vi "CEF_error generator.vi"(4 "concatenate (F)":bool, 5 "error (T)":bool=TRUE, 6 "error in":errorcluster, 7 "source":string="error generator.vi", 8 "append error message":string, 9 "error code (0)":i32) -> (0 "error out":errorcluster)   [LabVIEW 2025, in "CEF.lvlib"]
doc: "Converts an error or warning code to an error cluster. This VI is useful when you receive a return value from a shared library call or when you return user-defined error codes.Copyright 2017 National Instruments Corporation\n\nLicensed under the Apache License, Version 2.0 (the \"License\"); you may not use this file except in compliance with the License. You may obtain a copy of the License at http://www.apache.org/licenses/LICENSE-2.0\nUnless required by applicable law or agreed to in writing, software distributed under the License is distributed on an \"AS IS\" BASIS, WITHOUT WARRANTIES OR CONDITIONS OF ANY KIND, either express or implied. See the License for the specific language governing permissions and limitations under the License."
uses:
  CEF.lvlib
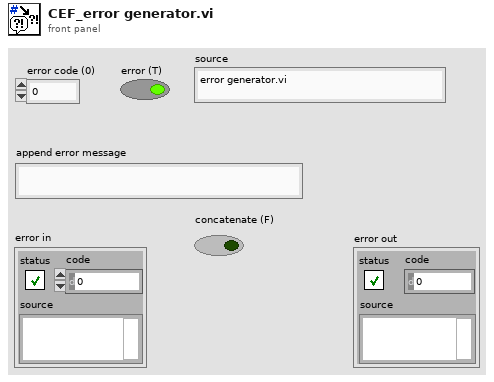
[diagram p1: front panel]
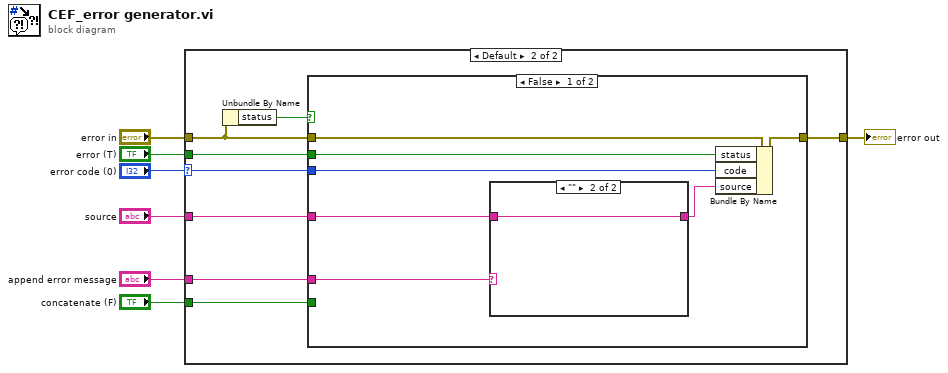
[diagram p0: block diagram]
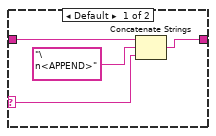
[diagram p3: hidden frame]
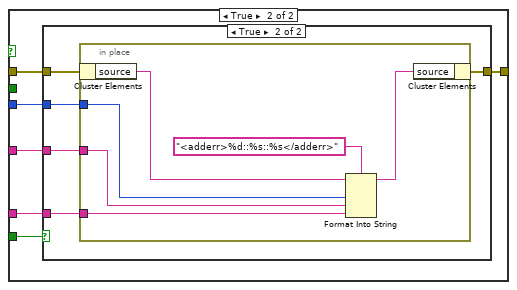
[diagram p4: hidden frame]
diagram:
  n1 = case shown="Default" "error code (0)" {
    selector: "error code (0)" -> [_ w15]
    tunnel: "error in" -> [w8 w11]
    tunnel: [w8 w16] -> w5
    tunnel: "source" -> [_ w14]
    tunnel: "append error message" -> [_ w13]
    tunnel: "error (T)" -> [_ w12]
    tunnel: "concatenate (F)" -> [_ w9]
    frame 0 {
      # "If the error code in equals zero, then propagate the error in cluster regardless of its value."
    }
    frame Default {
      n2 = Unbundle By Name(w11) -> ("status"=w10:bool)
      n3 = case shown="False" w10 {
        tunnel: [w22 w32] -> w16
        tunnel: w15 -> [w23 w31]
        tunnel: w14 -> [w19 w30]
        tunnel: w13 -> [w21 w29]
        tunnel: w12 -> [w18 _]
        tunnel: w11 -> [w17 w33]
        tunnel: w9 -> [_ w34]
        frame False {
          n4 = case shown="\"\"" w21 {
            selector: w21 -> [w25 _]
            tunnel: [w24 w28] -> w20
            tunnel: w19 -> [w27 w28]
            frame Default {
              n5 = Concatenate Strings(w27, "\n<APPEND>" ("string"), w25) -> (w24:string)
            }
            frame "" {
            }
          }
          n6 = Bundle By Name(cluster=w17, "status"=w18, "code"=w23, "source"=w20) -> (w22:errorcluster)
        }
        frame True {
          n7 = case shown="True" w34 {
            tunnel: w33 -> [w35 w40]
            tunnel: [w35 w39] -> w32
            tunnel: w31 -> [_ w38]
            tunnel: w30 -> [_ w37]
            tunnel: w29 -> [_ w36]
            frame False {
              # "An error in trumps any error code input."
            }
            frame True {
              n8 = in-place {
                in-place-border: w38 -> [w44]
                in-place-border: w37 -> [w43]
                in-place-border: w36 -> [w42]
                n9 = in-place-cluster #1(w40) -> ("source"=w46:string)
                n10 = Format Into String(format string="<adderr>%d::%s::%s</adderr>", initial string=w46, w44, w43, w42) -> (resulting string=w45:string)  [unwired: 1 in, 1 out]
                n11 = in-place-cluster #1("source"=w45) -> (w39:errorcluster)
              }
            }
          }
        }
      }
    }
  }
  "error out" <- w5
